vi "Lab Panel V5.22.1.vi"() -> ()   [LabVIEW 2013] (continued)
                          }
                        }
                        n3208 = local read "LAB05 TEMP"() -> (w5947:T12)
                        n3209 = local read "TEMP LA05"() -> (w5948:T9)
                        n3210 = call "sub vi - temperature delay v3.vi"("2-run"=w5929, "1-run"=w5930, "temp values IN"=w5948, "temp signals"=w5947) -> ("T2-N"=w5943:dbl, "T2-L"=w5944:dbl, "T1-N"=w5945:dbl, "T1-L"=w5946:dbl, "temp values OUT"=w5942:T44)  [unwired: 3 in]
                        n3211 = local write "TEMP LA05"(w5942) -> ()
                        n3212 = Unbundle By Name(w5957) -> ("1 (TL) cal"=w5949:dbl, "1 (TN) cal"=w5952:dbl, "2 (TL) cal"=w5951:dbl, "2 (TN) cal"=w5950:dbl)  [unwired: 6 out]
                        n3213 = Multiply(x=w5946, y=w5949) -> (x*y=w5938:dbl)
                        n3214 = Multiply(x=w5945, y=w5952) -> (x*y=w5937:dbl)
                        n3215 = Multiply(x=w5944, y=w5951) -> (x*y=w5934:dbl)
                        n3216 = Multiply(x=w5943, y=w5950) -> (x*y=w5933:dbl)
                        n3217 = case shown="True" w5929 {
                          tunnel: w5934 -> [w5959 w5964]
                          tunnel: w5939 -> [_ w5962]
                          tunnel: [w5959 w5963] -> w5932
                          tunnel: w5933 -> [w5958 w5961]
                          tunnel: [w5958 w5960] -> w5931
                          frame False {
                          }
                          frame True {
                            n3218 = Multiply(x=w5962, y=w5961) -> (x*y=w5960:dbl)
                            n3219 = Multiply(x=w5962, y=w5964) -> (x*y=w5963:dbl)
                          }
                        }
                        n3220 = case shown="True" w5930 {
                          tunnel: w5938 -> [w5966 w5971]
                          tunnel: w5939 -> [_ w5969]
                          tunnel: [w5966 w5970] -> w5936
                          tunnel: w5937 -> [w5965 w5968]
                          tunnel: [w5965 w5967] -> w5935
                          frame False {
                          }
                          frame True {
                            n3221 = Multiply(x=w5969, y=w5968) -> (x*y=w5967:dbl)
                            n3222 = Multiply(x=w5969, y=w5971) -> (x*y=w5970:dbl)
                          }
                        }
                        n3223 = local read "SIG LAB05-1"() -> (w5956:T2)
                        n3224 = Bundle By Name(cluster=w5956, "Tmp Live"=w5936, "Tmp Neut"=w5935) -> (w5955:T2)
                        n3225 = local read "SIG LAB05-2"() -> (w5954:T2)
                        n3226 = Bundle By Name(cluster=w5954, "Tmp Live"=w5932, "Tmp Neut"=w5931) -> (w5953:T2)
                        n3227 = local write "SIG LAB05-1"(w5955) -> ()
                        n3228 = local write "SIG LAB05-2"(w5953) -> ()
                      }
                    }
                  }
                }
              }
            }
          }
          frame #20 {
            # "write data to display panel"
            n3229 = global write "Global display 1.vi" "TEST 5-2"(w6008) -> ()
            n3230 = global write "Global display 1.vi" "TEST 4-2"(w6010) -> ()
            n3231 = global write "Global display 1.vi" "TEST 1-2"(w6016) -> ()
            n3232 = global write "Global display 1.vi" "TEST 3-1"(w6013) -> ()
            n3233 = global write "Global display 1.vi" "TEST 5-1"(w6009) -> ()
            n3234 = global write "Global display 1.vi" "TEST 1-1"(w6017) -> ()
            n3235 = global write "Global display 1.vi" "TEST 3-2"(w6012) -> ()
            n3236 = global write "Global display 1.vi" "TEST 4-1"(w6011) -> ()
            n3237 = global write "Global display 1.vi" "TEST 2-2"(w6014) -> ()
            n3238 = global write "Global display 1.vi" "TEST 2-1"(w6015) -> ()
            n3239 = global read "Global display 3.vi" "log 1-1"() -> (→"LOG LAB01-1":string)
            n3240 = global read "Global display 3.vi" "log 3-1"() -> (→"LOG LAB03-1":string)
            n3241 = global read "Global display 3.vi" "log 1-2"() -> (→"LOG LAB01-2":string)
            n3242 = property on="Tab Control 2" class="TabCtl (strict)"() -> ("Pages"=w6007:refnum<vi>[])  [unwired: 2 in, 2 out]
            n3243 = global read "Global display 3.vi" "log 2-1"() -> (→"LOG LAB02-1":string)
            n3244 = global read "Global display 3.vi" "log 2-2"() -> (→"LOG LAB02-2":string)
            n3245 = global read "Global display 3.vi" "log 4-2"() -> (→"LOG LAB04-2":string)
            n3246 = global read "Global display 3.vi" "log 5-2"() -> (→"LOG LAB05-2":string)
            n3247 = global read "Global display 3.vi" "log 5-1"() -> (→"LOG LAB05-1":string)
            n3248 = global read "Global display 3.vi" "log 4-1"() -> (→"LOG LAB04-1":string)
            n3249 = global read "Global display 3.vi" "log 3-2"() -> (→"LOG LAB03-2":string)
            n3250 = Index Array(array=w6007, index=8) -> (element=w6005:refnum<vi>)
            n3251 = property class="Page"(reference=w6005) -> ("PageVis"=w6004:bool)  [unwired: 1 in, 2 out]
            n3252 = global write "Global display 3.vi" "admin"(w6004) -> ()
            n3253 = local read "O/I  LAB05-2"() -> (w6058:bool)
            n3254 = local read "O/I  LAB05-1"() -> (w6059:bool)
            n3255 = local read "O/I  LAB03-2"() -> (w6062:bool)
            n3256 = local read "O/I  LAB04-2"() -> (w6060:bool)
            n3257 = local read "O/I  LAB04-1"() -> (w6061:bool)
            n3258 = local read "O/I  LAB03-1"() -> (w6063:bool)
            n3259 = local read "O/I  LAB01-2"() -> (w6066:bool)
            n3260 = local read "O/I  LAB01-1"() -> (w6067:bool)
            n3261 = local read "O/I  LAB02-1"() -> (w6065:bool)
            n3262 = local read "O/I  LAB02-2"() -> (w6064:bool)
            n3263 = global write "Global display 1.vi" "5-2 O/F"(w6058) -> ()
            n3264 = global write "Global display 1.vi" "5-1 O/F"(w6059) -> ()
            n3265 = global write "Global display 1.vi" "4-1 O/F"(w6061) -> ()
            n3266 = global write "Global display 1.vi" "4-2 O/F"(w6060) -> ()
            n3267 = global write "Global display 1.vi" "3-2 O/F"(w6062) -> ()
            n3268 = global write "Global display 1.vi" "3-1 O/F"(w6063) -> ()
            n3269 = global write "Global display 1.vi" "2-2 O/F"(w6064) -> ()
            n3270 = global write "Global display 1.vi" "2-1 O/F"(w6065) -> ()
            n3271 = global write "Global display 1.vi" "1-2 O/F"(w6066) -> ()
            n3272 = global write "Global display 1.vi" "1-1 O/F"(w6067) -> ()
            n3273 = local read "TEMP START LAB02-2"() -> (w5990:cluster{"TL":dbl, "TN":dbl})
            n3274 = local read "run lab05-2"() -> (w6048:bool)
            n3275 = local read "TEMP START LAB01-2"() -> (w5992:cluster{"TL":dbl, "TN":dbl})
            n3276 = local read "TEMP START LAB02-1"() -> (w5991:cluster{"TL":dbl, "TN":dbl})
            n3277 = local read "TEMP START LAB04-1"() -> (w5987:cluster{"TL":dbl, "TN":dbl})
            n3278 = local read "TEMP START LAB04-2"() -> (w5986:cluster{"TL":dbl, "TN":dbl})
            n3279 = local read "run lab04-1"() -> (w6051:bool)
            n3280 = local read "run lab04-2"() -> (w6050:bool)
            n3281 = local read "run lab05-1"() -> (w6049:bool)
            n3282 = local read "TEMP START LAB01-1"() -> (w5993:cluster{"TL":dbl, "TN":dbl})
            n3283 = local read "TEMP START LAB05-2"() -> (w5984:cluster{"TL":dbl, "TN":dbl})
            n3284 = local read "TEMP START LAB05-1"() -> (w5985:cluster{"TL":dbl, "TN":dbl})
            n3285 = local read "run lab03-2"() -> (w6052:bool)
            n3286 = local read "TEMP START LAB03-2"() -> (w5988:cluster{"TL":dbl, "TN":dbl})
            n3287 = local read "TEMP START LAB03-1"() -> (w5989:cluster{"TL":dbl, "TN":dbl})
            n3288 = local read "run lab02-1"() -> (w6055:bool)
            n3289 = local read "run lab03-1"() -> (w6053:bool)
            n3290 = local read "run lab01-2"() -> (w6056:bool)
            n3291 = local read "run lab02-2"() -> (w6054:bool)
            n3292 = local read "run lab01-1"() -> (w6057:bool)
            n3293 = global write "Global display 1.vi" "5-2 R/S"(w6048) -> ()
            n3294 = global write "Global display 1.vi" "5-1 R/S"(w6049) -> ()
            n3295 = global write "Global display 1.vi" "4-2 R/S"(w6050) -> ()
            n3296 = global write "Global display 1.vi" "4-1 R/S"(w6051) -> ()
            n3297 = global write "Global display 1.vi" "3-2 R/S"(w6052) -> ()
            n3298 = global write "Global display 1.vi" "1-2 R/S"(w6056) -> ()
            n3299 = global write "Global display 1.vi" "2-1 R/S"(w6055) -> ()
            n3300 = global write "Global display 1.vi" "3-1 R/S"(w6053) -> ()
            n3301 = global write "Global display 1.vi" "2-2 R/S"(w6054) -> ()
            n3302 = global write "Global display 1.vi" "1-1 R/S"(w6057) -> ()
            n3303 = global write "Global display 3.vi" "TEMP ST 05-2"(w5984) -> ()
            n3304 = global write "Global display 3.vi" "TEMP ST 05-1"(w5985) -> ()
            n3305 = global write "Global display 3.vi" "TEMP ST 03-2"(w5988) -> ()
            n3306 = global write "Global display 3.vi" "TEMP ST 04-2"(w5986) -> ()
            n3307 = global write "Global display 3.vi" "TEMP ST 01-1"(w5993) -> ()
            n3308 = global write "Global display 3.vi" "TEMP ST 01-2"(w5992) -> ()
            n3309 = global write "Global display 3.vi" "TEMP ST 04-1"(w5987) -> ()
            n3310 = global write "Global display 3.vi" "TEMP ST 02-1"(w5991) -> ()
            n3311 = global write "Global display 3.vi" "TEMP ST 02-2"(w5990) -> ()
            n3312 = global write "Global display 3.vi" "TEMP ST 03-1"(w5989) -> ()
            n3313 = local read "DISP LAB04-2"() -> (w6040:T4)
            n3314 = local read "DISP LAB05-1"() -> (w6039:T4)
            n3315 = local read "DISP LAB04-1"() -> (w6041:T4)
            n3316 = local read "DISP LAB05-2"() -> (w6038:T4)
            n3317 = local read "DISP LAB03-1"() -> (w6043:T4)
            n3318 = local read "DISP LAB03-2"() -> (w6042:T4)
            n3319 = local read "DISP LAB01-2"() -> (w6046:T4)
            n3320 = local read "DISP LAB02-1"() -> (w6045:T4)
            n3321 = local read "DISP LAB02-2"() -> (w6044:T4)
            n3322 = local read "DISP LAB01-1"() -> (w6047:T4)
            n3323 = local read "TEMP RISE LAB05-1"() -> (w5975:cluster{"TL":dbl, "TN":dbl})
            n3324 = local read "TEMP RISE LAB05-2"() -> (w5974:cluster{"TL":dbl, "TN":dbl})
            n3325 = local read "TEMP RISE LAB04-2"() -> (w5976:cluster{"TL":dbl, "TN":dbl})
            n3326 = local read "TEMP RISE LAB04-1"() -> (w5977:cluster{"TL":dbl, "TN":dbl})
            n3327 = local read "TEMP RISE LAB03-2"() -> (w5978:cluster{"TL":dbl, "TN":dbl})
            n3328 = local read "TEMP RISE LAB03-1"() -> (w5979:cluster{"TL":dbl, "TN":dbl})
            n3329 = local read "TEMP RISE LAB01-2"() -> (w5982:cluster{"TL":dbl, "TN":dbl})
            n3330 = local read "TEMP RISE LAB02-2"() -> (w5980:cluster{"TL":dbl, "TN":dbl})
            n3331 = local read "TEMP RISE LAB01-1"() -> (w5983:cluster{"TL":dbl, "TN":dbl})
            n3332 = local read "TEMP RISE LAB02-1"() -> (w5981:cluster{"TL":dbl, "TN":dbl})
            n3333 = global write "Global display 2.vi" "DISP LAB05-1"(w6039) -> ()
            n3334 = global write "Global display 2.vi" "DISP LAB05-2"(w6038) -> ()
            n3335 = global write "Global display 2.vi" "DISP LAB04-2"(w6040) -> ()
            n3336 = global write "Global display 2.vi" "DISP LAB02-1"(w6045) -> ()
            n3337 = global write "Global display 2.vi" "DISP LAB02-2"(w6044) -> ()
            n3338 = global write "Global display 2.vi" "DISP LAB04-1"(w6041) -> ()
            n3339 = global write "Global display 2.vi" "DISP LAB01-2"(w6046) -> ()
            n3340 = global write "Global display 2.vi" "DISP LAB01-1"(w6047) -> ()
            n3341 = global write "Global display 2.vi" "DISP LAB03-1"(w6043) -> ()
            n3342 = global write "Global display 2.vi" "DISP LAB03-2"(w6042) -> ()
            n3343 = global write "Global display 3.vi" "TEMP RS 05-2"(w5974) -> ()
            n3344 = global write "Global display 3.vi" "TEMP RS 05-1"(w5975) -> ()
            n3345 = global write "Global display 3.vi" "TEMP RS 03-2"(w5978) -> ()
            n3346 = global write "Global display 3.vi" "TEMP RS 02-1"(w5981) -> ()
            n3347 = global write "Global display 3.vi" "TEMP RS 02-2"(w5980) -> ()
            n3348 = global write "Global display 3.vi" "TEMP RS 04-2"(w5976) -> ()
            n3349 = global write "Global display 3.vi" "TEMP RS 01-2"(w5982) -> ()
            n3350 = global write "Global display 3.vi" "TEMP RS 03-1"(w5979) -> ()
            n3351 = global write "Global display 3.vi" "TEMP RS 04-1"(w5977) -> ()
            n3352 = global write "Global display 3.vi" "TEMP RS 01-1"(w5983) -> ()
            n3353 = local read "SET LAB05-2"() -> (w6028:T5)
            n3354 = local read "SET LAB05-1"() -> (w6029:T5)
            n3355 = local read "SET LAB04-1"() -> (w6031:T5)
            n3356 = local read "SET LAB04-2"() -> (w6030:T5)
            n3357 = local read "SET LAB03-1"() -> (w6033:T5)
            n3358 = local read "SET LAB03-2"() -> (w6032:T5)
            n3359 = local read "SET LAB02-2"() -> (w6034:T5)
            n3360 = local read "SET LAB01-2"() -> (w6036:T5)
            n3361 = local read "SET LAB02-1"() -> (w6035:T5)
            n3362 = local read "SET LAB01-1"() -> (w6037:T5)
            n3363 = global write "Global display 2.vi" "SET LAB05-2"(w6028) -> ()
            n3364 = global write "Global display 2.vi" "SET LAB05-1"(w6029) -> ()
            n3365 = global write "Global display 2.vi" "SET LAB04-1"(w6031) -> ()
            n3366 = global write "Global display 2.vi" "SET LAB04-2"(w6030) -> ()
            n3367 = global write "Global display 2.vi" "SET LAB03-2"(w6032) -> ()
            n3368 = global write "Global display 2.vi" "SET LAB02-2"(w6034) -> ()
            n3369 = global write "Global display 2.vi" "SET LAB03-1"(w6033) -> ()
            n3370 = global write "Global display 2.vi" "SET LAB01-2"(w6036) -> ()
            n3371 = global write "Global display 2.vi" "SET LAB01-1"(w6037) -> ()
            n3372 = global write "Global display 2.vi" "SET LAB02-1"(w6035) -> ()
            n3373 = local read "RESULT LAB01-1"() -> (w6027:bool)
            n3374 = local read "RESULT LAB03-2"() -> (w6022:bool)
            n3375 = local read "RESULT LAB04-1"() -> (w6021:bool)
            n3376 = local read "RESULT LAB04-2"() -> (w6020:bool)
            n3377 = local read "RESULT LAB02-2"() -> (w6024:bool)
            n3378 = local read "RESULT LAB01-2"() -> (w6026:bool)
            n3379 = local read "RESULT LAB02-1"() -> (w6025:bool)
            n3380 = local read "RESULT LAB03-1"() -> (w6023:bool)
            n3381 = local read "RESULT LAB05-1"() -> (w6019:bool)
            n3382 = local read "RESULT LAB05-2"() -> (w6018:bool)
            n3383 = global write "Global display 2.vi" "RESULT LAB05-1"(w6019) -> ()
            n3384 = global write "Global display 2.vi" "RESULT LAB01-2"(w6026) -> ()
            n3385 = global write "Global display 2.vi" "RESULT LAB03-2"(w6022) -> ()
            n3386 = global write "Global display 2.vi" "RESULT LAB04-1"(w6021) -> ()
            n3387 = global write "Global display 2.vi" "RESULT LAB04-2"(w6020) -> ()
            n3388 = global write "Global display 2.vi" "RESULT LAB05-2"(w6018) -> ()
            n3389 = global write "Global display 2.vi" "RESULT LAB03-1"(w6023) -> ()
            n3390 = global write "Global display 2.vi" "RESULT LAB02-1"(w6025) -> ()
            n3391 = global write "Global display 2.vi" "RESULT LAB02-2"(w6024) -> ()
            n3392 = global write "Global display 2.vi" "RESULT LAB01-1"(w6027) -> ()
          }
          frame #21 {
            # "simulate values"
            n3393 = global write "Global display 4.vi" "LAB deg C"("LAB deg C") -> ()
          }
          frame #22 {
            # "end main and display program"
            n3394 = stacked-sequence {
              seq-local: [_ w6072 _] -> [_ _ w6075]
              tunnel: w6069 -> [w6070 _ _]
              frame #0 {
                n3395 = case shown="True" w6070 {
                  frame False {
                  }
                  frame True {
                    n3396 = One Button Dialog(message="Excessive number of USB \nresets done, re-start program.") -> ()  [unwired: 1 in, 1 out]
                  }
                }
              }
              frame #1 {
                # "check for reset error"
                n3397 = local read "Reset Error"() -> (w6072:bool)
                n3398 = case shown="True" w6072 {
                  frame False {
                  }
                  frame True {
                    n3399 = One Button Dialog(message="USB Reset ERROR, program will be stopped.\nClose program, close windows, switch panel off\nand re power panel. If error persists seek help.") -> ()  [unwired: 1 in, 1 out]
                  }
                }
              }
              frame #2 {
                # "end labview session"
                n3400 = Or(x=w6075, y="stop all") -> (x .or. y?=w6074:bool)
                n3401 = Quit LabVIEW(quit? (T)=w6074) -> ()
                n3402 = global write "Global display 1.vi" "stop disp"(w6074) -> ()
              }
            }
          }
        }
        n3403 = node-c288() -> ()  [unwired: 1 in, 1 out]
        "loops" <- w335
      }
      n3404 = node-c288(w308) -> ()  [unwired: 1 out]
    }
  }
